vi "SaveZstack.vi"(6 "Scan Parameters":T2={"DAQ Resolution"=0.0, "AOD Parameters"={"Nvox"=0, "Zoom"=0, "Xc"=0.0, "Yc"=0.0, "Acceptance Angle"=0.0, "AOD Central Frequency"=0, "movex"=0.0, "movey"=0.0, "astig"=0.0, "p"=0.0, "Dwell Time"=0.0, "Z Position"=0.0, "xoma"=0.0, "xoda"=0.0, "yoma"=0.0, "yoda"=0.0, "Nx"=0.0, "msReduce"=0.0}, "Controls Cluster"={"Pockels Control"=0.019999999552965164, "PMT1"=0, "PMT2"=0, "No of Averages"=1, "Pockels"=37.243898882770964, "Back Aperture"=1.3556779193328632}}, 7 "Boolean":bool, 8 "Channelnames":string[](array[string])=["RedChannel", "GreenChannel"], 9 "zstack number":i32, 10 "ImageArray":T1[](array[typedef]), 11 "base path":path) -> ()   [LabVIEW 2017]
uses:
  <vilib>/vision/Image Controls.llb/IMAQ Image.ctl
  <vilib>/Utility/xml.llb/Write to XML File(string).vi
  <vilib>/vision/NI_Vision_Development_Module.lvlib
panel:
  out "Numeric":i32
  in  "S/W version":string="NeuroImageV4 is used for Data Acquisition"
  in  "ZRange":string
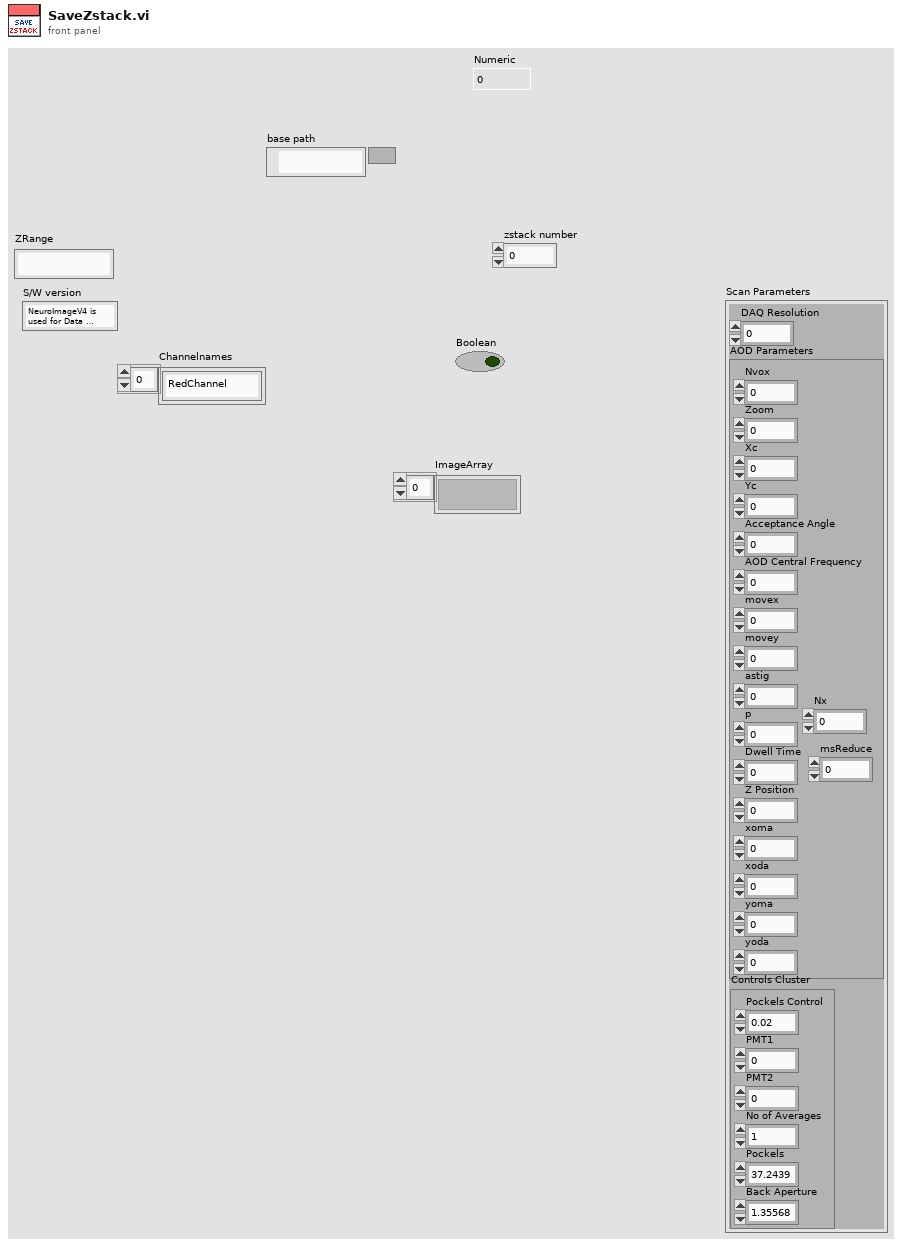
[diagram p1: front panel]
types:
  T1 = typedef "IMAQ Image.ctl" = refnum<image>
  T2 = cluster{"DAQ Resolution":dbl, "AOD Parameters":cluster{"Nvox":i16, "Zoom":i8, "Xc":dbl, "Yc":dbl, "Acceptance Angle":dbl, "AOD Central Frequency":i32, "movex":dbl, "movey":dbl, "astig":dbl, "p":dbl, "Dwell Time":dbl, "Z Position":sgl, "xoma":dbl, "xoda":dbl, "yoma":dbl, "yoda":dbl, "Nx":dbl, "msReduce":dbl}, "Controls Cluster":cluster{"Pockels Control":dbl, "PMT1":i32, "PMT2":i32, "No of Averages":i32, "Pockels":dbl, "Back Aperture":dbl}}
  T3 = typedef "Image Type" = u32
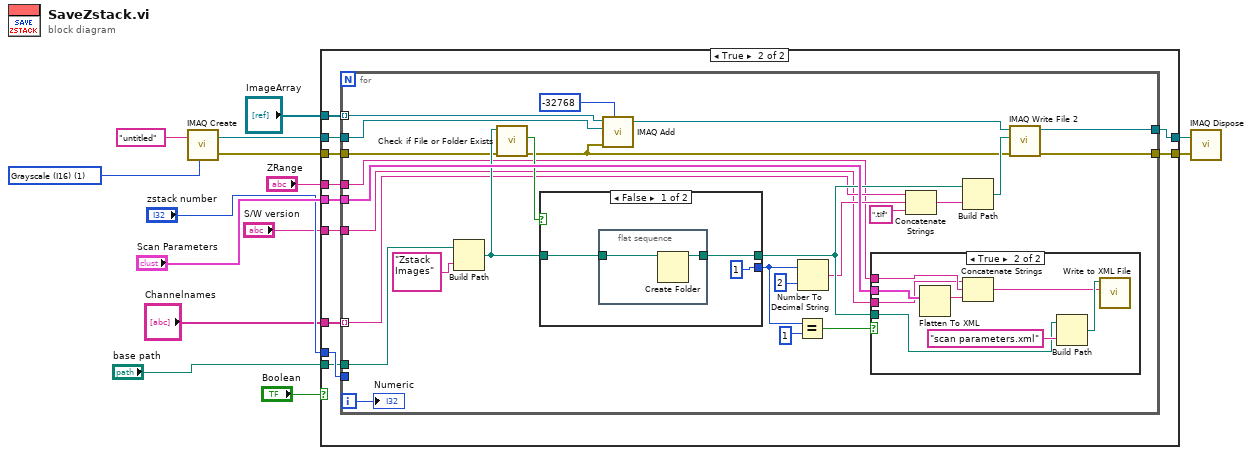
[diagram p0: block diagram]
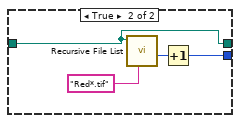
[diagram p4: hidden frame]
diagram:
  w10 = T3 1 items=["Grayscale (U8)", "Grayscale (I16)", "Grayscale (SGL)", "Complex (CSG)", "RGB (U32)", "HSL (U32)", "RGB (U64)"] ("Image Type")
  n1 = call "IMAQ Create"("Image Name"="untitled", "Image Type"=w10) -> ("New Image"=w9:T1, "error out"=w7:errorcluster)  [unwired: 3 in]
  n2 = case shown="True" "Boolean" {
    tunnel: "ImageArray" -> [_ w24]
    tunnel: "Scan Parameters" -> [_ w27]
    tunnel: "base path" -> [_ w18]
    tunnel: "zstack number" -> [_ w26]
    tunnel: w9 -> [w16 w25]
    tunnel: [w16 w23] -> w8
    tunnel: w7 -> [w15 w17]
    tunnel: [w15 w22] -> w6
    tunnel: "Channelnames" -> [_ w21]
    tunnel: "ZRange" -> [_ w20]
    tunnel: "S/W version" -> [_ w19]
    frame False {
    }
    frame True {
      n3 = for {
        tunnel: w27 -> [w53]
        tunnel: w26 -> [_]
        tunnel: w25 -> [w41]
        tunnel: w24 -> [w40] mode=indexing
        tunnel: [w38] -> w23
        tunnel: [w37] -> w22
        tunnel: w21 -> [w36] mode=indexing
        tunnel: w20 -> [w35]
        tunnel: w19 -> [w34]
        tunnel: w18 -> [w33]
        tunnel: w17 -> [w31]
        i -> [w28]
        n4 = Build Path(base path=w33, name or relative path="Zstack Images" ("string")) -> (appended path=w50:path)
        n5 = call <vilib>:"Check if File or Folder Exists.vi"("error in (no error)"=w31, "path"=w50) -> ("error out"=w30:errorcluster, "file or folder exists?"=w51:bool)  [unwired: 7 in, 1 out]
        n6 = case shown="False" w51 {
          tunnel: w50 -> [w64 w70]
          tunnel: [w63 w70] -> w52
          tunnel: [1 w67] -> w29
          frame False {
            n7 = flat-sequence {
              tunnel: [w65] -> w63
              tunnel: w64 -> [w66]
              frame #0 {
                n8 = Create Folder(path (use dialog)=w66) -> (created path=w65:path)  [unwired: 2 in, 2 out]
              }
            }
          }
          frame True {
            n9 = call <vilib>:"Recursive File List.vi"("pattern"="Red*.tif", "Folder Path"=w70) -> ("Number of Files"=w68:i32)  [unwired: 5 in, 4 out]
            n10 = Increment(x=w68) -> (x+1=w67:i32)
          }
        }
        n11 = call "IMAQ Add"("Image Src A"=w40, "Constant"=i16 -32768, "Image Dst"=w41, "error in (no error)"=w30) -> ("Image Dst Out"=w39:T1)  [unwired: 3 in, 1 out]
        n12 = Equal?(x=w29, y=1) -> (x = y?=w46:bool)
        n13 = Number To Decimal String(number=w29, width (-)=i16 2) -> (decimal integer string=w42:string)
        n14 = case shown="True" w46 {
          tunnel: w53 -> [_ w59]
          tunnel: w52 -> [_ w58]
          tunnel: w35 -> [_ w57]
          tunnel: w34 -> [_ w54]
          frame False {
          }
          frame True {
            n15 = Flatten To XML(anything=w59) -> (xml string=w56:string)
            n16 = Concatenate Strings(w54, w57, w56) -> (w55:string)
            n17 = Build Path(base path=w58, name or relative path="scan parameters.xml") -> (appended path=w60:path)
            n18 = call-poly <vilib>:"Write to XML File.vi"("XML Input"=w55, "XML File Path"=w60) -> ()  [unwired: 7 in, 3 out]
          }
        }
        n19 = Concatenate Strings(w36, w42, ".tif" ("string")) -> (w44:string)
        n20 = Build Path(base path=w52, name or relative path=w44) -> (appended path=w48:path)
        n21 = call-poly "IMAQ Write File 2"("error in (no error)"=w30, "File Path"=w48, "Image"=w39) -> ("error out"=w37:errorcluster, "Image Out (duplicate)"=w38:T1)  [unwired: 7 in]
        "Numeric" <- w28
      }
    }
  }
  n22 = call "IMAQ Dispose"("Image"=w8, "error in (no error)"=w6) -> ()  [unwired: 4 in, 1 out]
